vi "Get Value by Name.vi"(8 "error in (no error)":errorcluster, 10 "Name":string, 11 "Processing in":refnum<class "Processing.lvclass">) -> (0 "error out":errorcluster, 2 "Value":variant, 3 "Processing out":refnum<class "Processing.lvclass">)   [LabVIEW 2020, in "HTTP Server.lvlib" / "Processing.lvclass"]
uses:
  Processing.lvclass
  Values/Values.lvclass
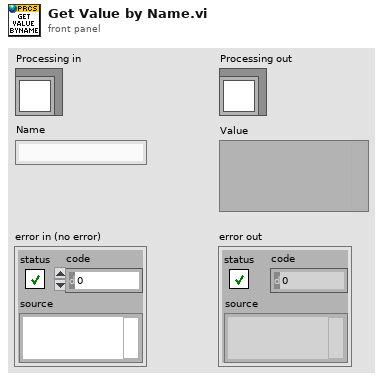
[diagram p1: front panel]
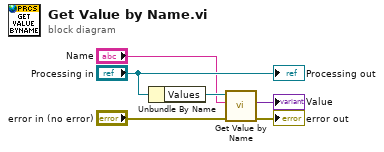
[diagram p0: block diagram]
diagram:
  n1 = Unbundle By Name("Processing in") -> ("Values"=w5:refnum<class "Values.lvclass">)
  n2 = call "Get Value by Name.vi"("error in (no error)"="error in (no error)", "Name"="Name", "Values in"=w5) -> ("error out"=→"error out":errorcluster, "Value"=→"Value":variant)  [unwired: 6 in, 1 out]
  "Processing out" <- "Processing in"
